vi "Elapsed Times Global.vi"() -> ()   [LabVIEW 2013]
panel:
  out "Elapsed Times":fxp<+,40,40>[](array[numeric]) format="%.30g"
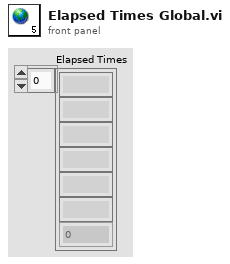
[diagram p1: front panel]
diagram:
